vi "Form Broadcast Log Text.vi"(10 "Data String Input":string, 11 "Broadcast":string) -> (3 "String to Write":string)   [LabVIEW 2015, in "Generic Module Library.lvlib" / "Template G_Module.lvlib"]
uses:
  Template G_Module.lvlib
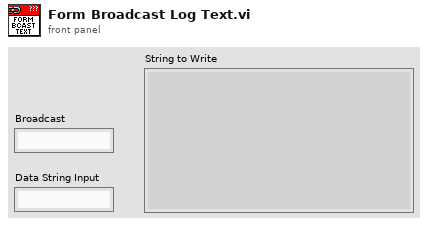
[diagram p1: front panel]
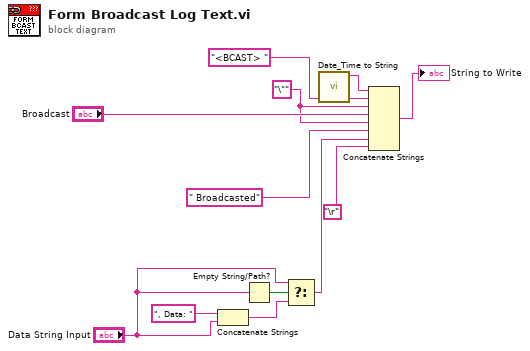
[diagram p0: block diagram]
diagram:
  w2 = "\"" ("string")
  n1 = Concatenate Strings(", Data: " ("string"), "Data String Input") -> (w11:string)
  n2 = Empty String/Path?(string/path="Data String Input") -> (empty?=w9:bool)
  n3 = Select(t="Data String Input", s=w9, f=w11) -> (s? t:f=w5:string)
  n4 = call "Date_Time to String.vi"() -> ("date/time string"=w8:string)  [unwired: 11 in]
  n5 = Concatenate Strings(w8, "<BCAST> " ("string"), w2, "Broadcast", w2, " Broadcasted" ("string"), w5, "\r") -> (→"String to Write":string)
